vi "calc sp go up.vi"(8 "error in (no error)":errorcluster, 11 "Stand in":refnum<class "Stand.lvclass">) -> (0 "error out":errorcluster)   [LabVIEW 2019, in "Stand.lvclass"]
uses:
  Stand.lvclass
  Stand.lvclass/Stand.ctl
  TypeDef/SP_TYPE.ctl
  c91f4351-afbf-4a48-b204-0d489dec29b1.vi
  50fb84da-4633-4161-b856-f10d1b653a37.vi
  Global/Global Constant.vi
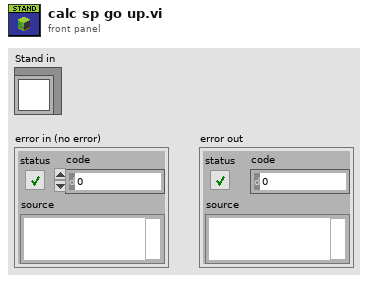
[diagram p1: front panel]
types:
  T1 = typedef "SP_TYPE.ctl" = enum16{"ERROR", "ZIRO", "BASE", "SP"}
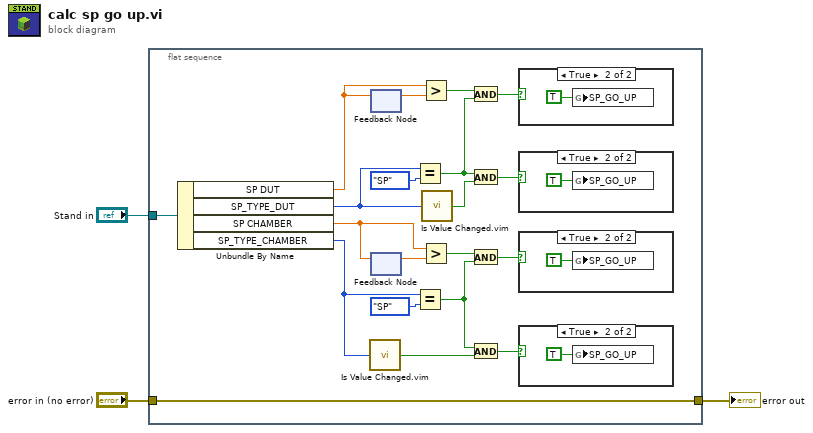
[diagram p0: block diagram]
diagram:
  n1 = flat-sequence {
    tunnel: "Stand in" -> [w23]
    tunnel: "error in (no error)" -> [w12]
    tunnel: [w12] -> w2
    frame #0 {
      n2 = Unbundle By Name(w23) -> ("SP DUT"=w17:dbl, "SP_TYPE_DUT"=w5:T1, "SP CHAMBER"=w19:dbl, "SP_TYPE_CHAMBER"=w11:T1)
      n3 = call "Is Value Changed.vim"("value"=w11) -> ("changed or first call?"=w10:bool)
      n4 = feedback #1() -> (w22:dbl)  [unwired: 1 in]
      n5 = feedback-in #1(w17) -> ()
      n6 = feedback #2() -> (w20:dbl)  [unwired: 1 in]
      n7 = feedback-in #2(w19) -> ()
      n8 = Equal?(x=w5, y=SP_TYPE."SP") -> (x = y?=w4:bool)
      n9 = Equal?(x=w11, y=SP_TYPE."SP") -> (x = y?=w9:bool)
      n10 = Greater?(x=w17, y=w22) -> (0:w21:bool)
      n11 = Greater?(x=w19, y=w20) -> (0:w18:bool)
      n12 = call "Is Value Changed.vim"("value"=w5) -> ("changed or first call?"=w6:bool)
      n13 = And(x=w21, y=w4) -> (x .and. y?=w13:bool)
      n14 = And(x=w4, y=w6) -> (x .and. y?=w7:bool)
      n15 = And(x=w18, y=w9) -> (x .and. y?=w15:bool)
      n16 = And(x=w9, y=w10) -> (x .and. y?=w8:bool)
      n17 = case shown="True" w13 {
        frame False {
        }
        frame True {
          n18 = global write "Global Constant.vi" "SP_GO_UP"(TRUE ("SP_GO_UP")) -> ()
        }
      }
      n19 = case shown="True" w7 {
        frame False {
        }
        frame True {
          n20 = global write "Global Constant.vi" "SP_GO_UP"(TRUE ("SP_GO_UP")) -> ()
        }
      }
      n21 = case shown="True" w15 {
        frame False {
        }
        frame True {
          n22 = global write "Global Constant.vi" "SP_GO_UP"(TRUE ("SP_GO_UP")) -> ()
        }
      }
      n23 = case shown="True" w8 {
        frame False {
        }
        frame True {
          n24 = global write "Global Constant.vi" "SP_GO_UP"(TRUE ("SP_GO_UP")) -> ()
        }
      }
    }
  }
  "error out" <- w2
